vi "read.vi"() -> ()   [LabVIEW 2015]
uses:
  <vilib>/Instr/_visa.llb/VISA Configure Serial Port (Instr).vi
panel:
  out "concatenated string":string
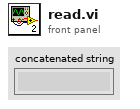
[diagram p1: front panel]
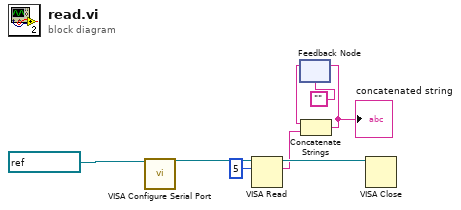
[diagram p0: block diagram]
diagram:
  n1 = call-poly "VISA Configure Serial Port"("VISA resource name"=refnum<visa-resource-name> "COM13") -> ("VISA resource name out"=w7:refnum<visa-resource-name>)  [unwired: 13 in, 1 out]
  n2 = VISA Read(VISA resource name=w7, byte count=u32 5) -> (VISA resource name out=w5:refnum<visa-resource-name>, read buffer=w4:string)  [unwired: 1 in, 2 out]
  n3 = feedback #1("") -> (w2:string)
  n4 = Concatenate Strings(w2, w4) -> (w3:string)
  "concatenated string" <- w3
  n5 = feedback-in #1(w3) -> ()
  n6 = VISA Close(VISA resource name=w5) -> ()  [unwired: 1 in, 1 out]
